vi "pulse_generator_multiheater_refnum.vi"(1 "125W Fixed/Variable":refnum<vi>, 2 "Stop! Refnum":refnum<vi>, 3 "Pulse Generator Control Multiheater Refnums":T1) -> ()   [LabVIEW 2015]
uses:
  <vilib>/Utility/error.llb/DialogType.ctl
  <vilib>/DAQmx/create/channels.llb/DAQmx Create Channel (DO-Digital Output).vi
  <vilib>/DAQmx/configure/timing.llb/DAQmx Timing (Implicit).vi
  <vilib>/DAQmx/create/channels.llb/DAQmx Create Channel (CO-Pulse Generation-Frequency).vi
  <resource>/objmgr/daqmx.rc
  <vilib>/DAQmx/write.llb/DAQmx Write (Digital 1D Bool NChan 1Samp 1Line).vi
  <vilib>/DAQmx/write.llb/DAQmx Write (Digital Bool 1Line 1Point).vi
  pulse_generator_controls_multiheater_refnums.ctl
panel:
  out "Stopped!":bool caption="OK"
  in  "Stop! Local":bool
  out "message":string=" INSTRUCTIONS:\r\rNormal Use:  When using subVIs that incorporate the error in/error out (or error I/O) structure, place this handler where you want to inform the user of an error, typically at the end of the I/O data path, as the last action of the program.  If the error in error? is ERROR, the handler creates a message describing the error and its source.  If the type of dialog = 1 (default), the message is displayed to the user, who can only acknowedge it.  If the type = 2, the user can acknowledge the message or abort execution; aborting a program with active I/O is not recommended.  If the type = 0, no message is displayed; this is used to process the error programmatically, and the error out cluster elements are wired to individual terminals for that reason.  \r\rOther Use:\n\r\nlocal testing.  To test the error code of a subVI or function that does not have the error I/O structure, you can wire its error code and a source string to the local error code and error source inputs.  If error in error? indicates no error and error code is not equal to 0, the local code and source are substituted for the error in values, and error? is set TRUE (ERROR)."
  in  "SwitchHelper":bool
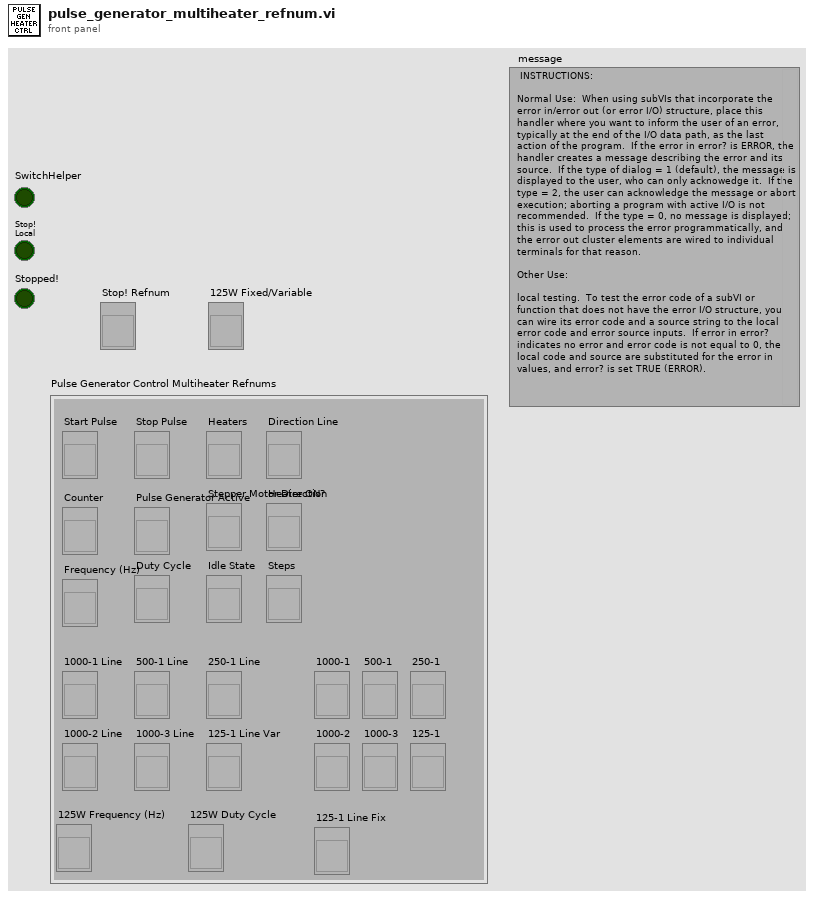
[diagram p1: front panel]
types:
  T1 = typedef "pulse_generator_controls_multiheater_refnums.ctl" = cluster{"Start Pulse":refnum<vi>, "Stop Pulse":refnum<vi>, "Heaters":refnum<vi>, "Counter":refnum<vi>, "Frequency (Hz)":refnum<vi>, "Duty Cycle":refnum<vi>, "Idle State":refnum<vi>, "Pulse Generator Active":refnum<vi>, "Stepper Motor Direction":refnum<vi>, "Steps":refnum<vi>, "Direction Line":refnum<vi>, "1000-1 Line":refnum<vi>, "1000-2 Line":refnum<vi>, "1000-3 Line":refnum<vi>, "500-1 Line":refnum<vi>, "250-1 Line":refnum<vi>, "125-1 Line Var":refnum<vi>, "1000-1":refnum<vi>, "1000-2":refnum<vi>, "1000-3":refnum<vi>, "500-1":refnum<vi>, "250-1":refnum<vi>, "125-1":refnum<vi>, "125W Frequency (Hz)":refnum<vi>, "125W Duty Cycle":refnum<vi>, "Heater ON?":refnum<vi>, "125-1 Line Fix":refnum<vi>}
  T2 = enum8{"Enabled", "Disabled", "Disabled and Grayed Out"}
  T3 = typedef "DialogType.ctl" = u16
  T4 = cluster{"1000-1":refnum<vi>, "1000-2":refnum<vi>, "1000-3":refnum<vi>, "500-1":refnum<vi>}
  T5 = cluster{"1000-1 Line":refnum<vi>, "1000-2 Line":refnum<vi>, "1000-3 Line":refnum<vi>, "500-1 Line":refnum<vi>, "250-1 Line":refnum<vi>}
  T6 = cluster{"1000-1 Line":refnum<vi>, "1000-2 Line":refnum<vi>, "1000-3 Line":refnum<vi>, "500-1 Line":refnum<vi>}
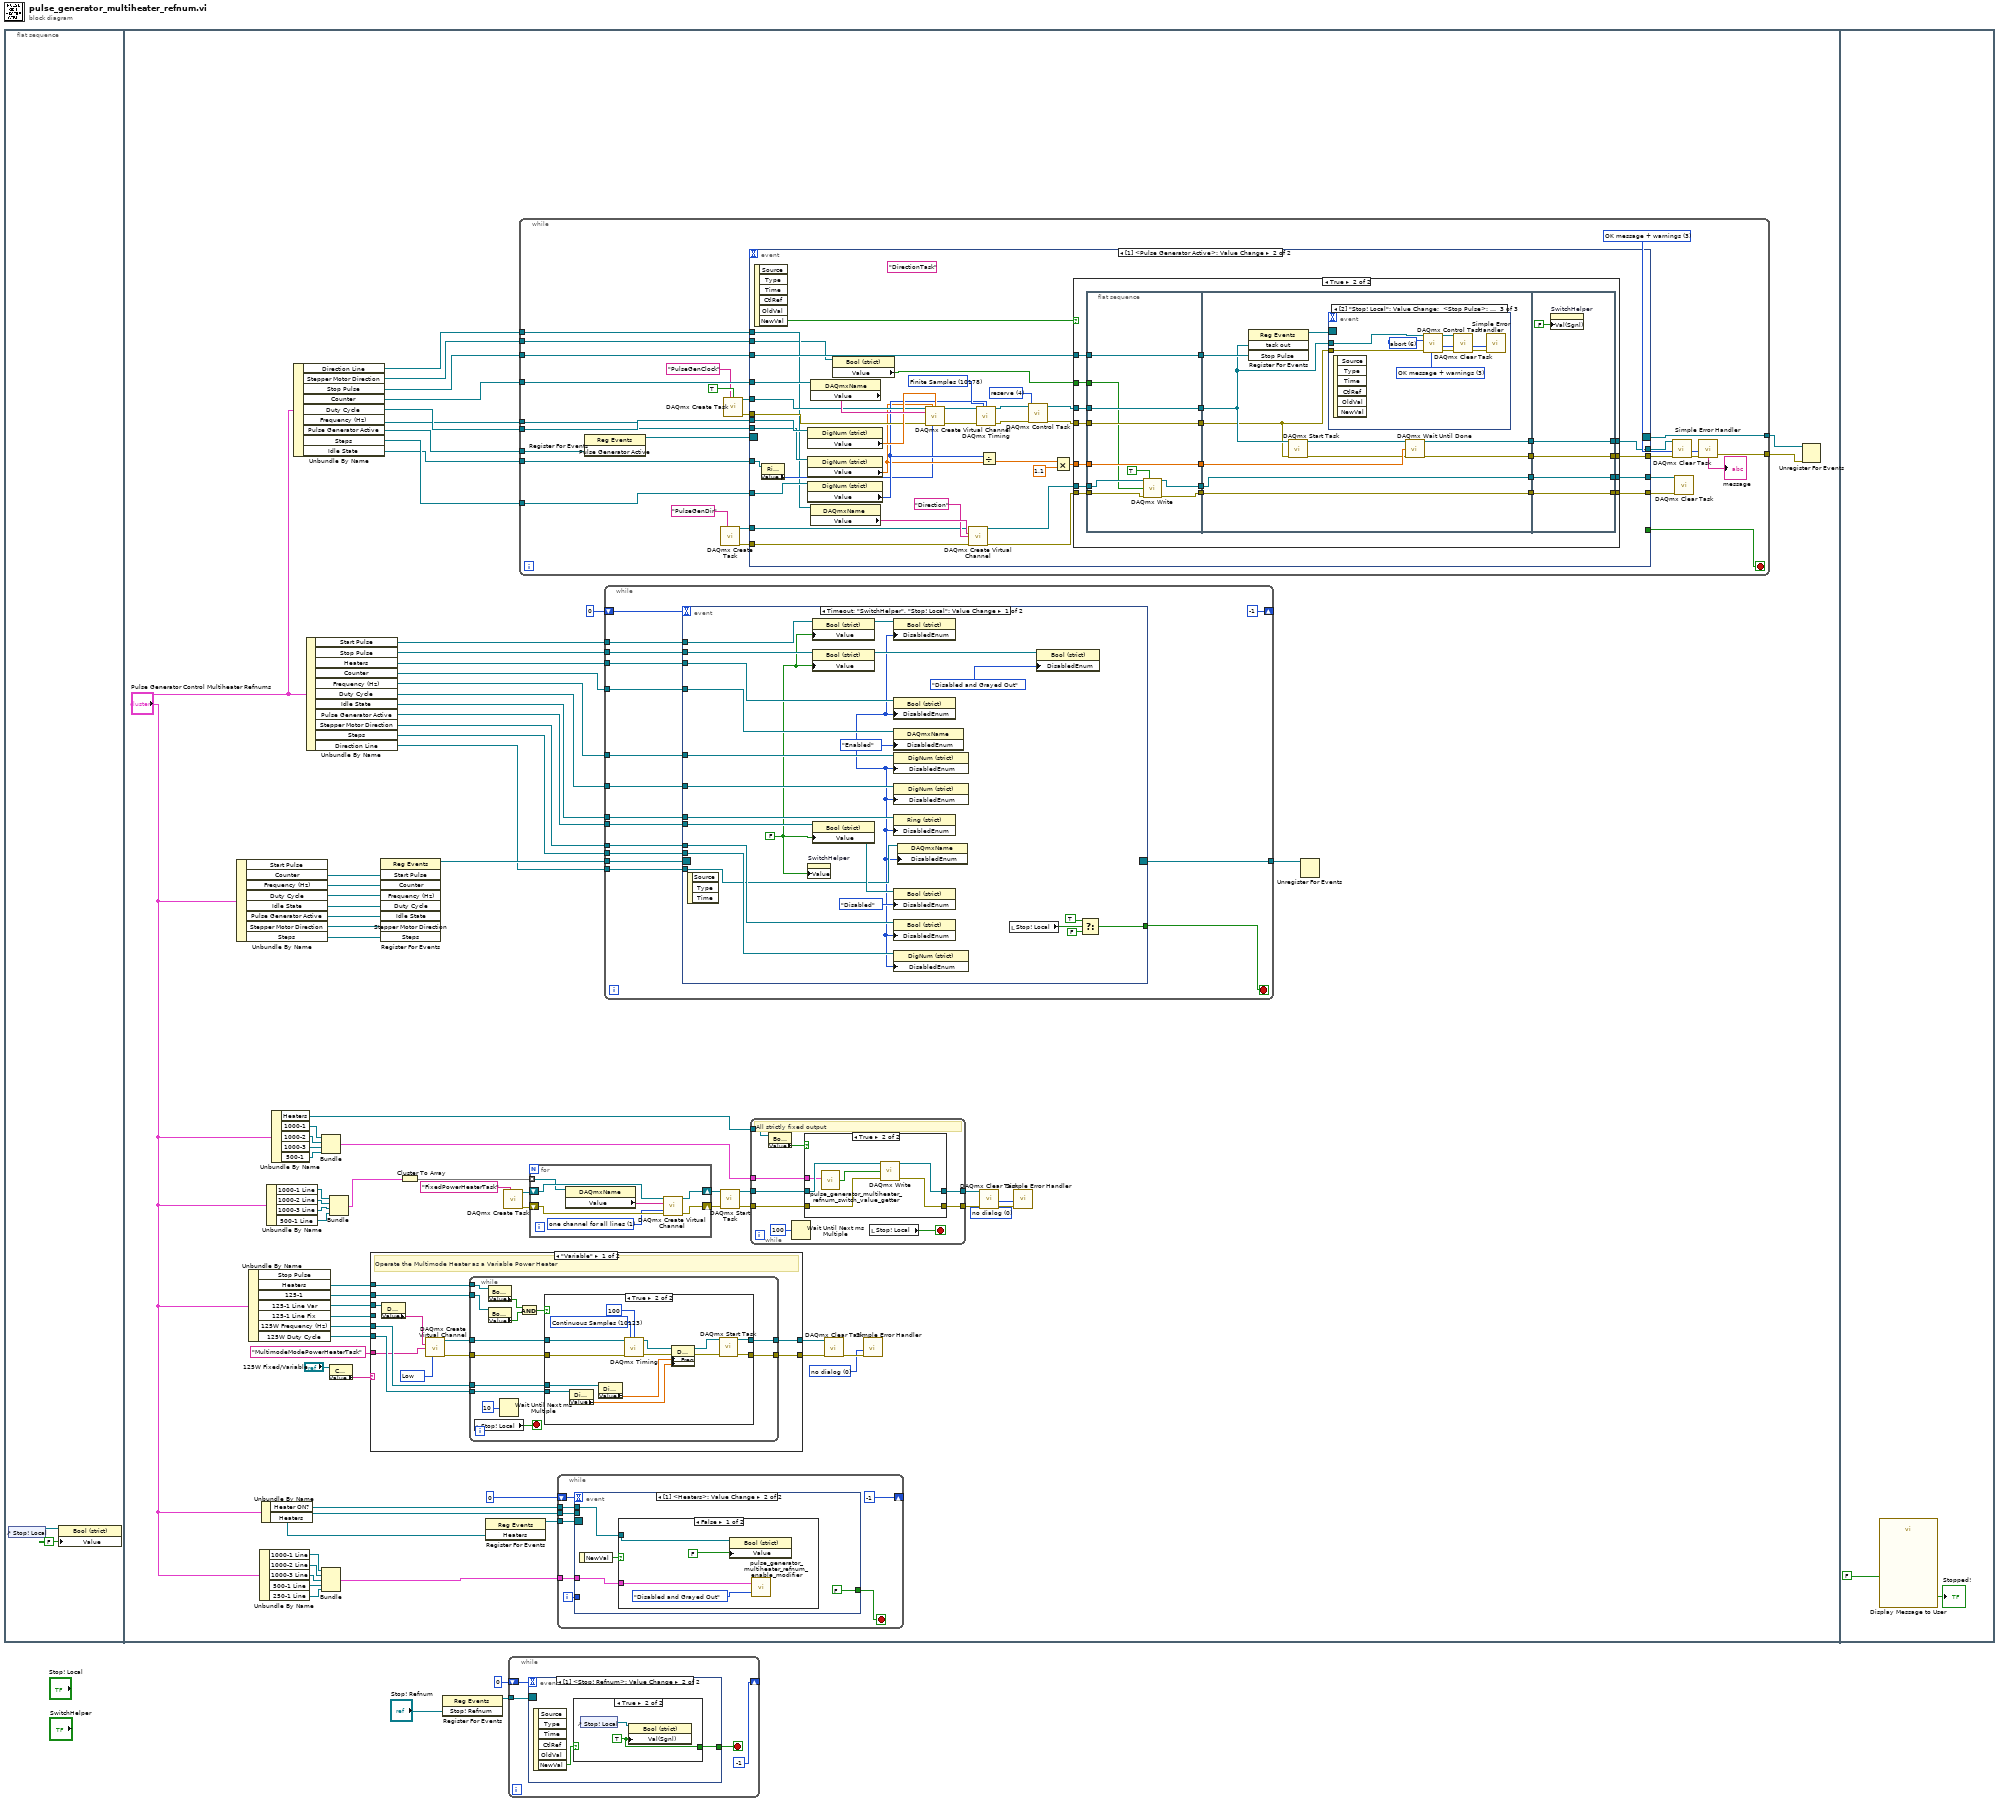
[diagram p0: block diagram]
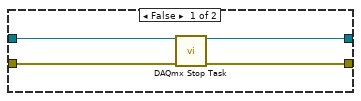
[diagram p2: hidden frame]
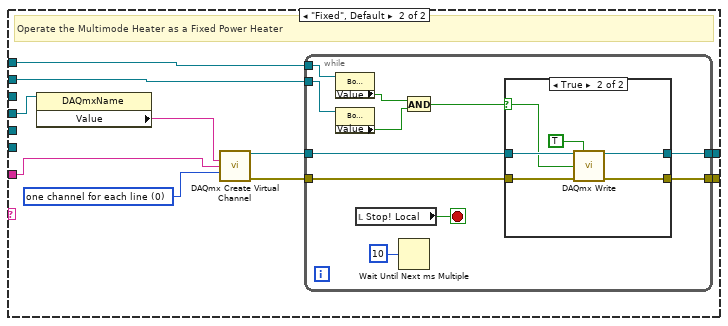
[diagram p3: hidden frame]
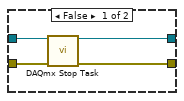
[diagram p4: hidden frame]
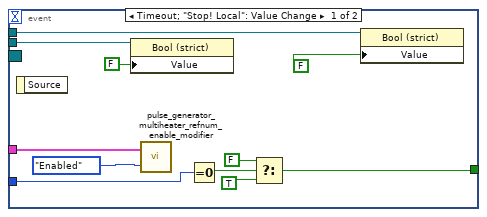
[diagram p5: hidden frame]
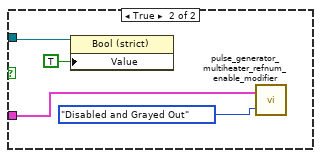
[diagram p6: hidden frame]
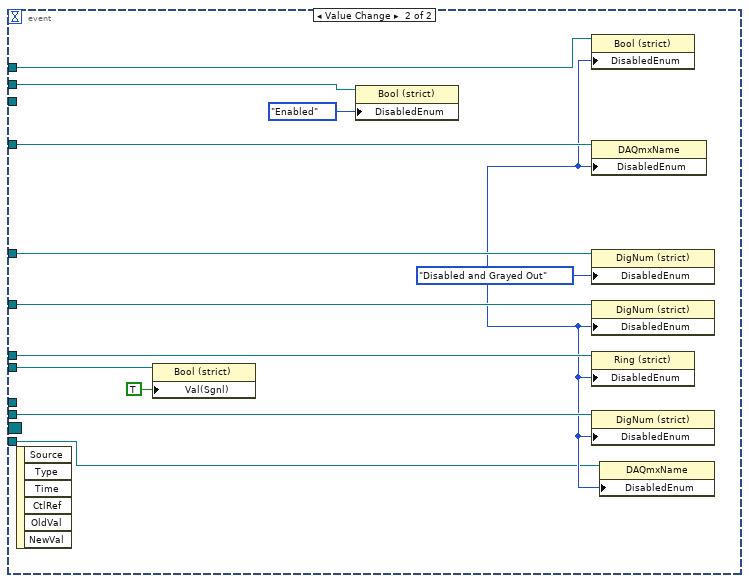
[diagram p8: hidden frame]
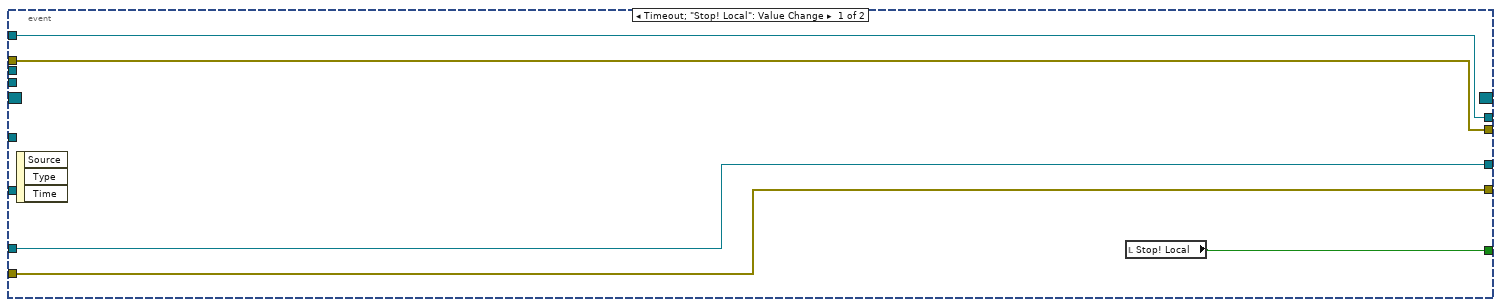
[diagram p9: hidden frame]
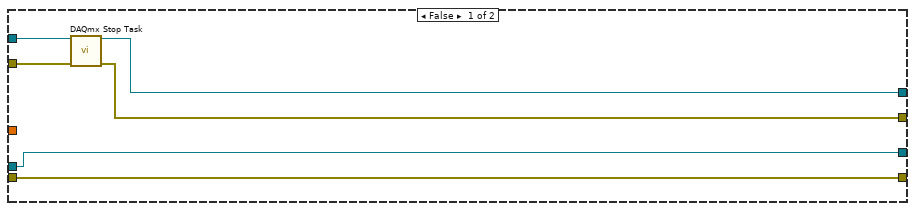
[diagram p10: hidden frame]
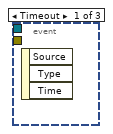
[diagram p11: hidden frame]
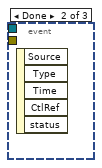
[diagram p12: hidden frame]
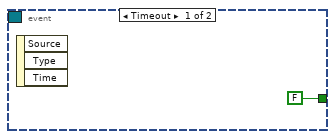
[diagram p13: hidden frame]
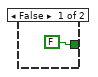
[diagram p14: hidden frame]
diagram:
  n1 = flat-sequence {
    frame #0 {
      n2 = control-ref of="Stop! Local"() -> (w4:refnum<vi>)
      n3 = property class="Bool (strict)"(reference=w4, "Value"=FALSE) -> ()  [unwired: 1 in, 2 out]
    }
    frame #1 {
      w7 = T3 0 items=["no dialog", "OK message", "continue or stop message", "OK message + warnings", "continue/stop + warnings"] ("type of dialog (OK msg:1)")
      w64 = T3 0 items=["no dialog", "OK message", "continue or stop message", "OK message + warnings", "continue/stop + warnings"] ("type of dialog (OK msg:1)")
      n4 = Unbundle By Name("Pulse Generator Control Multiheater Refnums") -> ("Start Pulse"=w73:refnum<vi>, "Counter"=w82:refnum<vi>, "Frequency (Hz)"=w81:refnum<vi>, "Duty Cycle"=w80:refnum<vi>, "Idle State"=w79:refnum<vi>, "Stepper Motor Direction"=w76:refnum<vi>, "Steps"=w75:refnum<vi>)  [unwired: 1 out]
      n5 = Unbundle By Name("Pulse Generator Control Multiheater Refnums") -> ("Heaters"=w14:refnum<vi>, "125-1"=w26:refnum<vi>, "125-1 Line Var"=w30:refnum<vi>, "125-1 Line Fix"=w8:refnum<vi>, "125W Frequency (Hz)"=w28:refnum<vi>, "125W Duty Cycle"=w27:refnum<vi>)  [unwired: 1 out]
      n6 = Unbundle By Name("Pulse Generator Control Multiheater Refnums") -> ("1000-1 Line"=w59:refnum<vi>, "1000-2 Line"=w58:refnum<vi>, "1000-3 Line"=w57:refnum<vi>, "500-1 Line"=w56:refnum<vi>, "250-1 Line"=w22:refnum<vi>)
      n7 = Unbundle By Name("Pulse Generator Control Multiheater Refnums") -> ("Heater ON?"=w62:refnum<vi>, "Heaters"=w50:refnum<vi>)
      n8 = Unbundle By Name("Pulse Generator Control Multiheater Refnums") -> ("1000-1 Line"=w20:refnum<vi>, "1000-2 Line"=w19:refnum<vi>, "1000-3 Line"=w18:refnum<vi>, "500-1 Line"=w17:refnum<vi>)
      n9 = Unbundle By Name("Pulse Generator Control Multiheater Refnums") -> ("Heaters"=w49:refnum<vi>, "1000-1"=w48:refnum<vi>, "1000-2"=w47:refnum<vi>, "1000-3"=w46:refnum<vi>, "500-1"=w45:refnum<vi>)
      n10 = Unbundle By Name("Pulse Generator Control Multiheater Refnums") -> ("Direction Line"=w12:refnum<vi>, "Stepper Motor Direction"=w11:refnum<vi>, "Stop Pulse"=w43:refnum<vi>, "Counter"=w39:refnum<vi>, "Duty Cycle"=w40:refnum<vi>, "Frequency (Hz)"=w37:refnum<vi>, "Pulse Generator Active"=w35:refnum<vi>, "Steps"=w33:refnum<vi>, "Idle State"=w29:refnum<vi>)
      n11 = Unbundle By Name("Pulse Generator Control Multiheater Refnums") -> ("Start Pulse"=w83:refnum<vi>, "Stop Pulse"=w42:refnum<vi>, "Heaters"=w60:refnum<vi>, "Counter"=w38:refnum<vi>, "Frequency (Hz)"=w36:refnum<vi>, "Duty Cycle"=w41:refnum<vi>, "Idle State"=w74:refnum<vi>, "Pulse Generator Active"=w34:refnum<vi>, "Stepper Motor Direction"=w66:refnum<vi>, "Steps"=w32:refnum<vi>, "Direction Line"=w13:refnum<vi>)
      n12 = Bundle("1000-1"=w48, "1000-2"=w47, "1000-3"=w46, "500-1"=w45) -> (w44:T4)  [unwired: 1 in]
      n13 = Bundle("1000-1 Line"=w59, "1000-2 Line"=w58, "1000-3 Line"=w57, "500-1 Line"=w56, "250-1 Line"=w22) -> (w16:T5)  [unwired: 1 in]
      n14 = Bundle("1000-1 Line"=w20, "1000-2 Line"=w19, "1000-3 Line"=w18, "500-1 Line"=w17) -> (w15:T6)  [unwired: 1 in]
      n15 = property class="CmbBox"(reference="125W Fixed/Variable") -> ("Value"=w9:string)  [unwired: 1 in, 2 out]
      n16 = case shown="\"Variable\"" w9 {
        tunnel: w30 -> [w96 _]
        tunnel: w28 -> [w91 _]
        tunnel: w27 -> [w90 _]
        tunnel: w26 -> [w89 w134]
        tunnel: [w88 w133] -> w24
        tunnel: [w87 w132] -> w23
        tunnel: w14 -> [w86 w131]
        tunnel: w8 -> [_ w130]
        tunnel: "MultimodeModePowerHeaterTask" ("new task name") -> [w85 w128]
        frame "Variable" {
          w94 = 10214 items=["High"=10192, "Low"=10214] ("idle state")
          # "Operate the Multimode Heater as a Variable Power Heater"
          n17 = property class="DAQmxName"(reference=w96) -> ("Value"=w95:string)  [unwired: 1 in, 2 out]
          n18 = call-poly <vilib>:"DAQmx Create Virtual Channel.vi"("counter"=w95, "name to assign"=w85, "idle state"=w94) -> ("task out"=w93:refnum<k21>, "error out"=w92:errorcluster)  [unwired: 11 in]
          n19 = while {
            tunnel: w93 -> [w107]
            tunnel: w92 -> [w106]
            tunnel: w89 -> [w101]
            tunnel: w91 -> [w105]
            tunnel: w90 -> [w104]
            tunnel: [w103] -> w88
            tunnel: [w102] -> w87
            tunnel: w86 -> [w100]
            stop <- w109 stop-if-true
            n20 = local read "Stop! Local"() -> (w109:bool)
            n21 = property class="Bool (strict)"(reference=w100) -> ("Value"=w98:bool)  [unwired: 1 in, 2 out]
            n22 = property class="Bool (strict)"(reference=w101) -> ("Value"=w97:bool)  [unwired: 1 in, 2 out]
            n23 = Wait Until Next ms Multiple(millisecond multiple=u32 10) -> ()  [unwired: 1 out]
            n24 = And(x=w98, y=w97) -> (x .and. y?=w99:bool)
            n25 = case shown="True" w99 {
              tunnel: w107 -> [w111 w127]
              tunnel: w106 -> [w110 w126]
              tunnel: w105 -> [_ w119]
              tunnel: w104 -> [_ w118]
              tunnel: [w113 w114] -> w103
              tunnel: [w112 w115] -> w102
              frame False {
                n26 = call <vilib>:"DAQmx Stop Task.vi"("task/channels in"=w111, "error in"=w110) -> ("task out"=w113:refnum<k21>, "error out"=w112:errorcluster)  [unwired: 12 in]
              }
              frame True {
                w125 = 10123 items=["Finite Samples"=10178, "Continuous Samples"=10123, "Hardware Timed Single Point"=12522] ("sample mode")
                n27 = property class="DigNum (strict)"(reference=w118) -> ("Value"=w120:dbl)  [unwired: 1 in, 2 out]
                n28 = property class="DigNum (strict)"(reference=w119) -> ("Value"=w121:dbl)  [unwired: 1 in, 2 out]
                n29 = call-poly <vilib>:"DAQmx Timing.vi"("task/channels in"=w127, "sample mode"=w125, "samples per channel"=100, "error in"=w126) -> ("task out"=w123:refnum<k21>, "error out"=w122:errorcluster)  [unwired: 10 in]
                n30 = property class="DAQmx Channel"(reference=w123, error in=w122, "CO.Pulse.Freq"=w121, "CO.Pulse.DutyCyc"=w120) -> (reference out=w117:refnum<k21>, error out=w116:errorcluster)
                n31 = call <vilib>:"DAQmx Start Task.vi"("task/channels in"=w117, "error in"=w116) -> ("task out"=w114:refnum<k21>, "error out"=w115:errorcluster)  [unwired: 12 in]
              }
            }
          }
        }
        frame "Fixed", Default {
          w129 = 0 items=["one channel for each line", "one channel for all lines"] ("line grouping")
          # "Operate the Multimode Heater as a Fixed Power Heater"
          n32 = property class="DAQmxName"(reference=w130) -> ("Value"=w137:string)  [unwired: 1 in, 2 out]
          n33 = call-poly <vilib>:"DAQmx Create Virtual Channel.vi"("lines"=w137, "name to assign"=w128, "line grouping"=w129) -> ("task out"=w136:refnum<k21>, "error out"=w135:errorcluster)  [unwired: 11 in]
          n34 = while {
            tunnel: w136 -> [w146]
            tunnel: w135 -> [w145]
            tunnel: w134 -> [w142]
            tunnel: [w144] -> w133
            tunnel: [w143] -> w132
            tunnel: w131 -> [w141]
            stop <- w148 stop-if-true
            n35 = property class="Bool (strict)"(reference=w141) -> ("Value"=w139:bool)  [unwired: 1 in, 2 out]
            n36 = property class="Bool (strict)"(reference=w142) -> ("Value"=w138:bool)  [unwired: 1 in, 2 out]
            n37 = local read "Stop! Local"() -> (w148:bool)
            n38 = Wait Until Next ms Multiple(millisecond multiple=u32 10) -> ()  [unwired: 1 out]
            n39 = And(x=w139, y=w138) -> (x .and. y?=w140:bool)
            n40 = case shown="True" w140 {
              selector: w140 -> [_ w153]
              tunnel: w146 -> [w150 w155]
              tunnel: w145 -> [w149 w154]
              tunnel: [w152 w158] -> w144
              tunnel: [w151 w157] -> w143
              frame False {
                n41 = call <vilib>:"DAQmx Stop Task.vi"("task/channels in"=w150, "error in"=w149) -> ("task out"=w152:refnum<k21>, "error out"=w151:errorcluster)  [unwired: 12 in]
              }
              frame True {
                n42 = call-poly <vilib>:"DAQmx Write.vi"("task/channels in"=w155, "auto start"=TRUE, "data"=w153, "error in"=w154) -> ("task out"=w158:refnum<k21>, "error out"=w157:errorcluster)  [unwired: 9 in, 1 out]
              }
            }
          }
        }
      }
      n43 = register-events(w73, w82, w81, w80, w79, w76, w75) -> (reference out=w78:refnum<event-registration>)  [unwired: 2 in, 1 out]
      n44 = Cluster To Array(cluster=w15) -> (array=w31:refnum<vi>[])
      n45 = register-events(w50) -> (reference out=w61:refnum<event-registration>)  [unwired: 2 in, 1 out]
      n46 = call <vilib>:"DAQmx Create Task.vi"("new task name"="FixedPowerHeaterTask") -> ("task out"=w53:refnum<k21>, "error out"=w52:errorcluster)  [unwired: 13 in]
      n47 = while {
        tunnel: w35 -> [w285]
        tunnel: [w287] -> w65
        tunnel: w33 -> [w280]
        tunnel: w40 -> [w278]
        tunnel: w37 -> [w275]
        tunnel: w39 -> [w279]
        tunnel: w43 -> [w286]
        tunnel: [w273] -> w63
        tunnel: w29 -> [w271]
        tunnel: w12 -> [w270]
        tunnel: w11 -> [w269]
        stop <- w274 stop-if-true
        w282 = T3 3 items=["no dialog", "OK message", "continue or stop message", "OK message + warnings", "continue/stop + warnings"] ("type of dialog (OK msg:1)")
        n48 = register-events(w285) -> (reference out=w284:refnum<event-registration>)  [unwired: 2 in, 1 out]
        n49 = call <vilib>:"DAQmx Create Task.vi"("new task name"="PulseGenDir") -> ("task out"=w268:refnum<k21>, "error out"=w267:errorcluster)  [unwired: 13 in]
        n50 = call <vilib>:"DAQmx Create Task.vi"("new task name"="PulseGenClock", "auto cleanup"=TRUE) -> ("task out"=w277:refnum<k21>, "error out"=w276:errorcluster)  [unwired: 12 in]
        n51 = event shown="[1] <Pulse Generator Active>: Value Change" {
          selector: w284 -> [_ _]
          dyn-events: [_ _] -> w287
          timeout: _ -> [_ _]
          tunnel: [w294 w331] -> w289
          tunnel: [w295 w332] -> w288
          tunnel: w277 -> [w295 w320]
          tunnel: w276 -> [w294 w319]
          tunnel: w286 -> [_ w330]
          tunnel: w280 -> [_ w325]
          tunnel: w279 -> [_ w323]
          tunnel: w278 -> [_ w321]
          tunnel: w275 -> [_ w316]
          tunnel: [w293 _] -> w274
          tunnel: w271 -> [_ w315]
          tunnel: w270 -> [_ w313]
          tunnel: w269 -> [_ w310]
          tunnel: w268 -> [w292 w308]
          tunnel: w267 -> [w291 w307]
          tunnel: [w292 w306] -> w266
          tunnel: [w291 w305] -> w265
          event Timeout; "Stop! Local": Value Change {
            n52 = event-data() -> ()  [unwired: 1 in, 3 out]
            n53 = local read "Stop! Local"() -> (w293:bool)
          }
          event Value Change {
            w302 = 4 items=["verify"=2, "reserve"=4, "commit"=3, "unreserve"=5, "abort"=6] ("action")
            (unwired) "DirectionTask" ("name to assign")
            w329 = 10178 items=["Finite Samples"=10178, "Continuous Samples"=10123, "Hardware Timed Single Point"=12522] ("sample mode")
            n54 = event-data() -> ("NewVal"=w333:bool)  [unwired: 1 in, 5 out]
            n55 = property class="Ring (strict)"(reference=w315) -> ("Value"=w314:i32)  [unwired: 1 in, 2 out]
            n56 = property class="DigNum (strict)"(reference=w321) -> ("Value"=w322:dbl)  [unwired: 1 in, 2 out]
            n57 = property class="DigNum (strict)"(reference=w316) -> ("Value"=w317:dbl)  [unwired: 1 in, 2 out]
            n58 = property class="DigNum (strict)"(reference=w325) -> ("Value"=w318:i32)  [unwired: 1 in, 2 out]
            n59 = property class="DAQmxName"(reference=w313) -> ("Value"=w312:string)  [unwired: 1 in, 2 out]
            n60 = property class="DAQmxName"(reference=w323) -> ("Value"=w324:string)  [unwired: 1 in, 2 out]
            n61 = property class="Bool (strict)"(reference=w310) -> ("Value"=w309:bool)  [unwired: 1 in, 2 out]
            n62 = call-poly <vilib>:"DAQmx Create Virtual Channel.vi"("task in"=w320, "frequency"=w317, "duty cycle"=w322, "counter"=w324, "error in"=w319, "idle state"=w314) -> ("task out"=w304:refnum<k21>, "error out"=w303:errorcluster)  [unwired: 8 in]
            n63 = call-poly <vilib>:"DAQmx Create Virtual Channel.vi"("task in"=w308, "lines"=w312, "name to assign"="Direction", "error in"=w307) -> ("task out"=w297:refnum<k21>, "error out"=w296:errorcluster)  [unwired: 10 in]
            n64 = call-poly <vilib>:"DAQmx Timing.vi"("task/channels in"=w304, "sample mode"=w329, "samples per channel"=w318, "error in"=w303) -> ("task out"=w301:refnum<k21>, "error out"=w300:errorcluster)  [unwired: 10 in]
            n65 = Divide(x=w318, y=w317) -> (x/y=w327:dbl)
            n66 = call <vilib>:"DAQmx Control Task.vi"("task/channels in"=w301, "action"=w302, "error in"=w300) -> ("task out"=w298:refnum<k21>, "error out"=w299:errorcluster)  [unwired: 11 in]
            n67 = Multiply(x=w327, y=1.1) -> (x*y=w326:dbl)
            n68 = case shown="True" w333 {
              tunnel: w298 -> [w339 w357]
              tunnel: w299 -> [w338 w360]
              tunnel: [w336 w359] -> w332
              tunnel: [w337 w358] -> w331
              tunnel: w330 -> [_ w354]
              tunnel: w326 -> [_ w353]
              tunnel: w309 -> [_ w352]
              tunnel: w297 -> [w335 w351]
              tunnel: w296 -> [w334 w350]
              tunnel: [w335 w348] -> w306
              tunnel: [w334 w346] -> w305
              frame False {
                n69 = call <vilib>:"DAQmx Stop Task.vi"("task/channels in"=w339, "error in"=w338) -> ("task out"=w336:refnum<k21>, "error out"=w337:errorcluster)  [unwired: 12 in]
              }
              frame True {
                n70 = flat-sequence {
                  tunnel: w350 -> [w365]
                  tunnel: w351 -> [w366]
                  tunnel: w352 -> [w361]
                  tunnel: w353 -> [w367]
                  tunnel: w354 -> [w368]
                  tunnel: w357 -> [w369]
                  tunnel: w360 -> [w370]
                  tunnel: [w370] -> w345
                  tunnel: [w369] -> w344
                  tunnel: [w368] -> w343
                  tunnel: [w367] -> w342
                  tunnel: [w364] -> w341
                  tunnel: [w363] -> w340
                  tunnel: [w381] -> w356
                  tunnel: [w380] -> w355
                  tunnel: [w371] -> w349
                  tunnel: [w372] -> w347
                  tunnel: w345 -> [w375]
                  tunnel: w344 -> [w376]
                  tunnel: w343 -> [w378]
                  tunnel: w342 -> [w377]
                  tunnel: w341 -> [w372]
                  tunnel: w340 -> [w371]
                  tunnel: [w392] -> w358
                  tunnel: [w393] -> w359
                  tunnel: w356 -> [w393]
                  tunnel: w355 -> [w392]
                  tunnel: w349 -> [w390]
                  tunnel: [w390] -> w348
                  tunnel: w347 -> [w389]
                  tunnel: [w389] -> w346
                  frame #0 {
                    n71 = call-poly <vilib>:"DAQmx Write.vi"("task/channels in"=w366, "auto start"=TRUE, "data"=w361, "error in"=w365) -> ("task out"=w363:refnum<k21>, "error out"=w364:errorcluster)  [unwired: 9 in, 1 out]
                  }
                  frame #1 {
                    n72 = register-events(w376, w378) -> (reference out=w379:refnum<event-registration>)  [unwired: 2 in, 1 out]
                    n73 = call <vilib>:"DAQmx Start Task.vi"("task/channels in"=w376, "error in"=w375) -> ("task out"=w374:refnum<k21>, "error out"=w373:errorcluster)  [unwired: 12 in]
                    n74 = event shown="[2] \"Stop! Local\": Value Change;  <Stop Pulse>: Value Change" {
                      selector: w379 -> [_ _ _]
                      dyn-events: _ -> [_ _ _]
                      timeout: _ -> [_ _ _]
                      tunnel: w376 -> [_ _ w388]
                      tunnel: w375 -> [_ _ w387]
                      event Timeout {
                        n75 = event-data() -> ()  [unwired: 1 in, 3 out]
                      }
                      event Done {
                        n76 = event-data() -> ()  [unwired: 1 in, 5 out]
                      }
                      event "Stop! Local": Value Change {
                        w382 = T3 3 items=["no dialog", "OK message", "continue or stop message", "OK message + warnings", "continue/stop + warnings"] ("type of dialog (OK msg:1)")
                        w386 = 6 items=["verify"=2, "reserve"=4, "commit"=3, "unreserve"=5, "abort"=6] ("action")
                        n77 = event-data() -> ()  [unwired: 1 in, 6 out]
                        n78 = call <vilib>:"DAQmx Control Task.vi"("task/channels in"=w388, "action"=w386, "error in"=w387) -> ("task out"=w385:refnum<k21>, "error out"=w384:errorcluster)  [unwired: 11 in]
                        n79 = call <vilib>:"DAQmx Clear Task.vi"("task in"=w385, "error in"=w384) -> ("error out"=w383:errorcluster)  [unwired: 13 in]
                        n80 = call <vilib>:"Simple Error Handler.vi"("type of dialog (OK msg:1)"=w382, "error in (no error)"=w383) -> ()  [unwired: 3 in, 5 out]
                      }
                    }
                    n81 = call <vilib>:"DAQmx Wait Until Done.vi"("task/channels in"=w374, "timeout (sec)"=w377, "error in"=w373) -> ("task out"=w381:refnum<k21>, "error out"=w380:errorcluster)  [unwired: 11 in]
                  }
                  frame #2 {
                    n82 = property on="SwitchHelper" class="Bool (strict)"("Val(Sgnl)"=FALSE ("Value (Signaling)")) -> ()  [unwired: 2 in, 2 out]
                  }
                }
              }
            }
          }
        }
        n83 = call <vilib>:"DAQmx Clear Task.vi"("task in"=w288, "error in"=w289) -> ("error out"=w290:errorcluster)  [unwired: 13 in]
        n84 = call <vilib>:"DAQmx Clear Task.vi"("task in"=w266, "error in"=w265) -> ()  [unwired: 13 in, 1 out]
        n85 = call <vilib>:"Simple Error Handler.vi"("type of dialog (OK msg:1)"=w282, "error in (no error)"=w290) -> ("error out"=w273:errorcluster, "message"=→"message":string)  [unwired: 3 in, 3 out]
      }
      n86 = for {
        tunnel: w31 -> [w161] mode=indexing
        shift-right: [w165] -> w55
        shift-left: w53 -> [w163]
        shift-right: [w164] -> w54
        shift-left: w52 -> [w162]
        w159 = 1 items=["one channel for each line", "one channel for all lines"] ("line grouping")
        n87 = property class="DAQmxName"(reference=w161) -> ("Value"=w160:string)  [unwired: 1 in, 2 out]
        n88 = call-poly <vilib>:"DAQmx Create Virtual Channel.vi"("task in"=w163, "lines"=w160, "line grouping"=w159, "error in"=w162) -> ("task out"=w165:refnum<k21>, "error out"=w164:errorcluster)  [unwired: 10 in]
      }
      n89 = while {
        tunnel: w61 -> [w173]
        shift-right: [-1 ("millisecond multiple")] -> _
        shift-left: 0 ("millisecond multiple") -> [w172]
        tunnel: w50 -> [w170]
        tunnel: w62 -> [w167]
        tunnel: w16 -> [w166]
        i -> [w169]
        stop <- w168 stop-if-true
        n90 = event shown="[1] <Heaters>: Value Change" {
          selector: w173 -> [_ _]
          dyn-events: _ -> [_ _]
          timeout: w172 -> [_ _]
          tunnel: w170 -> [w184 _]
          tunnel: w169 -> [w181 _]
          tunnel: [w178 FALSE ("f")] -> w168
          tunnel: w167 -> [w176 w187]
          tunnel: w166 -> [w175 w185]
          event Timeout; "Stop! Local": Value Change {
            n91 = event-data() -> ()  [unwired: 1 in, 1 out]
            n92 = property class="Bool (strict)"(reference=w184, "Value"=FALSE) -> ()  [unwired: 1 in, 2 out]
            n93 = call "pulse_generator_multiheater_refnum_enable_modifier.vi"("Disabled"=T2."Enabled", "DAQmxName Refnums"=w175) -> ()  [unwired: 1 in]
            n94 = Equal To 0?(x=w181) -> (x = 0?=w182:bool)
            n95 = Select(t=FALSE, s=w182, f=TRUE) -> (s? t:f=w178:bool)
            n96 = property class="Bool (strict)"(reference=w176, "Value"=FALSE) -> ()  [unwired: 1 in, 2 out]
          }
          event Value Change {
            n97 = event-data() -> ("NewVal"=w188:bool)  [unwired: 1 in]
            n98 = case shown="False" w188 {
              tunnel: w187 -> [w192 w195]
              tunnel: w185 -> [w190 w194]
              frame False {
                n99 = property class="Bool (strict)"(reference=w192, "Value"=FALSE) -> ()  [unwired: 1 in, 2 out]
                n100 = call "pulse_generator_multiheater_refnum_enable_modifier.vi"("Disabled"=T2."Disabled and Grayed Out", "DAQmxName Refnums"=w190) -> ()  [unwired: 1 in]
              }
              frame True {
                n101 = property class="Bool (strict)"(reference=w195, "Value"=TRUE) -> ()  [unwired: 1 in, 2 out]
                n102 = call "pulse_generator_multiheater_refnum_enable_modifier.vi"("Disabled"=T2."Disabled and Grayed Out", "DAQmxName Refnums"=w194) -> ()  [unwired: 1 in]
              }
            }
          }
        }
      }
      n103 = while {
        shift-right: [-1] -> _
        shift-left: 0 -> [w229]
        tunnel: w83 -> [w227]
        tunnel: w42 -> [w226]
        tunnel: w60 -> [w216]
        tunnel: w38 -> [w222]
        tunnel: w36 -> [w221]
        tunnel: w41 -> [w220]
        tunnel: w74 -> [w219]
        tunnel: w34 -> [w225]
        tunnel: w66 -> [w218]
        tunnel: w78 -> [w224]
        tunnel: [w223] -> w77
        tunnel: w32 -> [w217]
        tunnel: w13 -> [w214]
        stop <- w215 stop-if-true
        n104 = event shown="[0] Timeout;  \"SwitchHelper\", \"Stop! Local\": Value Change" {
          selector: w224 -> [_ _]
          dyn-events: [_ _] -> w223
          timeout: w229 -> [_ _]
          tunnel: w227 -> [w251 w263]
          tunnel: w226 -> [w250 w257]
          tunnel: w225 -> [w249 w255]
          tunnel: w222 -> [w238 w262]
          tunnel: w221 -> [w240 w258]
          tunnel: w220 -> [w242 w261]
          tunnel: w219 -> [w243 w260]
          tunnel: w218 -> [w237 _]
          tunnel: w217 -> [w241 w259]
          tunnel: w216 -> [w239 _]
          tunnel: [w234 _] -> w215
          tunnel: w214 -> [w231 w252]
          event Timeout; "SwitchHelper", "Stop! Local": Value Change {
            w230 = T2."Enabled" ("Disabled")
            w236 = FALSE ("Value")
            n105 = event-data() -> ()  [unwired: 1 in, 3 out]
            n106 = property on="SwitchHelper" class="Bool (strict)"("Value"=w236) -> ()  [unwired: 2 in, 2 out]
            n107 = property class="Bool (strict)"(reference=w251, "Value"=w236) -> (reference out=w248:refnum<vi>)  [unwired: 1 in, 1 out]
            n108 = property class="Bool (strict)"(reference=w250, "Value"=w236) -> (reference out=w247:refnum<vi>)  [unwired: 1 in, 1 out]
            n109 = property class="Bool (strict)"(reference=w249, "Value"=w236) -> (reference out=w246:refnum<vi>)  [unwired: 1 in, 1 out]
            n110 = property class="Bool (strict)"(reference=w248, "DisabledEnum"=w230) -> ()  [unwired: 1 in, 2 out]
            n111 = property class="Bool (strict)"(reference=w239, "DisabledEnum"=w230) -> ()  [unwired: 1 in, 2 out]
            n112 = property class="DAQmxName"(reference=w238, "DisabledEnum"=w230) -> ()  [unwired: 1 in, 2 out]
            n113 = property class="DigNum (strict)"(reference=w240, "DisabledEnum"=w230) -> ()  [unwired: 1 in, 2 out]
            n114 = property class="DigNum (strict)"(reference=w242, "DisabledEnum"=w230) -> ()  [unwired: 1 in, 2 out]
            n115 = property class="Ring (strict)"(reference=w243, "DisabledEnum"=w230) -> ()  [unwired: 1 in, 2 out]
            n116 = property class="Bool (strict)"(reference=w246, "DisabledEnum"=T2."Disabled" ("Disabled")) -> ()  [unwired: 1 in, 2 out]
            n117 = property class="Bool (strict)"(reference=w237, "DisabledEnum"=w230) -> ()  [unwired: 1 in, 2 out]
            n118 = property class="DigNum (strict)"(reference=w241, "DisabledEnum"=w230) -> ()  [unwired: 1 in, 2 out]
            n119 = property class="DAQmxName"(reference=w231, "DisabledEnum"=w230) -> ()  [unwired: 1 in, 2 out]
            n120 = local read "Stop! Local"() -> (w235:bool)
            n121 = property class="Bool (strict)"(reference=w247, "DisabledEnum"=T2."Disabled and Grayed Out" ("Disabled")) -> ()  [unwired: 1 in, 2 out]
            n122 = Select(t=TRUE ("Value"), s=w235, f=FALSE ("Value")) -> (s? t:f=w234:bool)
          }
          event Value Change {
            w253 = T2."Disabled and Grayed Out" ("Disabled")
            n123 = event-data() -> ()  [unwired: 1 in, 6 out]
            n124 = property class="Bool (strict)"(reference=w255, "Val(Sgnl)"=TRUE ("Value")) -> ()  [unwired: 1 in, 2 out]
            n125 = property class="Bool (strict)"(reference=w257, "DisabledEnum"=T2."Enabled" ("Disabled")) -> ()  [unwired: 1 in, 2 out]
            n126 = property class="Bool (strict)"(reference=w263, "DisabledEnum"=w253) -> ()  [unwired: 1 in, 2 out]
            n127 = property class="DAQmxName"(reference=w262, "DisabledEnum"=w253) -> ()  [unwired: 1 in, 2 out]
            n128 = property class="DigNum (strict)"(reference=w258, "DisabledEnum"=w253) -> ()  [unwired: 1 in, 2 out]
            n129 = property class="DigNum (strict)"(reference=w261, "DisabledEnum"=w253) -> ()  [unwired: 1 in, 2 out]
            n130 = property class="Ring (strict)"(reference=w260, "DisabledEnum"=w253) -> ()  [unwired: 1 in, 2 out]
            n131 = property class="DigNum (strict)"(reference=w259, "DisabledEnum"=w253) -> ()  [unwired: 1 in, 2 out]
            n132 = property class="DAQmxName"(reference=w252, "DisabledEnum"=w253) -> ()  [unwired: 1 in, 2 out]
          }
        }
      }
      n133 = call <vilib>:"DAQmx Start Task.vi"("task/channels in"=w55, "error in"=w54) -> ("task out"=w71:refnum<k21>, "error out"=w72:errorcluster)  [unwired: 12 in]
      n134 = while {
        tunnel: w71 -> [w203]
        tunnel: w72 -> [w202]
        tunnel: w49 -> [w198]
        tunnel: [w201] -> w70
        tunnel: [w200] -> w69
        tunnel: w44 -> [w199]
        stop <- w204 stop-if-true
        # "All strictly fixed output"
        n135 = property class="Bool (strict)"(reference=w198) -> ("Value"=w197:bool)  [unwired: 1 in, 2 out]
        n136 = Wait Until Next ms Multiple(millisecond multiple=u32 100) -> ()  [unwired: 1 out]
        n137 = case shown="True" w197 {
          tunnel: w203 -> [w207 w212]
          tunnel: w202 -> [w206 w209]
          tunnel: [w207 w213] -> w201
          tunnel: [w206 w208] -> w200
          tunnel: w199 -> [_ w211]
          frame False {
          }
          frame True {
            n138 = call "pulse_generator_multiheater_refnum_switch_value_getter.vi"("output cluster"=w211) -> ("Array"=w210:bool[])
            n139 = call-poly <vilib>:"DAQmx Write.vi"("task/channels in"=w212, "data"=w210, "error in"=w209) -> ("task out"=w213:refnum<k21>, "error out"=w208:errorcluster)  [unwired: 10 in, 1 out]
          }
        }
        n140 = local read "Stop! Local"() -> (w204:bool)
      }
      n141 = call <vilib>:"DAQmx Clear Task.vi"("task in"=w24, "error in"=w23) -> ("error out"=w25:errorcluster)  [unwired: 13 in]
      n142 = call <vilib>:"Simple Error Handler.vi"("type of dialog (OK msg:1)"=w7, "error in (no error)"=w25) -> ()  [unwired: 3 in, 5 out]
      n143 = call <vilib>:"DAQmx Clear Task.vi"("task in"=w70, "error in"=w69) -> ("error out"=w68:errorcluster)  [unwired: 13 in]
      n144 = call <vilib>:"Simple Error Handler.vi"("type of dialog (OK msg:1)"=w64, "error in (no error)"=w68) -> ()  [unwired: 3 in, 5 out]
      n145 = Unregister For Events(event registration refnum=w77) -> ()  [unwired: 1 in, 1 out]
      n146 = Unregister For Events(event registration refnum=w65, error in=w63) -> ()  [unwired: 1 out]
    }
    frame #2 {
      n147 = call "Display Message to User"("Enable"=FALSE) -> ("OK"=→"Stopped!":bool)  [unwired: 9 in, 1 out]
    }
  }
  n148 = register-events("Stop! Refnum") -> (reference out=w2:refnum<event-registration>)  [unwired: 2 in, 1 out]
  n149 = while {
    tunnel: w2 -> [w399]
    shift-right: [-1] -> _
    shift-left: 0 -> [w398]
    stop <- w396 stop-if-true
    n150 = event shown="[1] <Stop! Refnum>: Value Change" {
      selector: w399 -> [_ _]
      dyn-events: _ -> [_ _]
      timeout: w398 -> [_ _]
      tunnel: [FALSE ("Value (Signaling)") w401] -> w396
      event Timeout {
        n151 = event-data() -> ()  [unwired: 1 in, 3 out]
      }
      event Value Change {
        n152 = event-data() -> ("NewVal"=w402:bool)  [unwired: 1 in, 5 out]
        n153 = case shown="True" w402 {
          tunnel: [FALSE ("Value (Signaling)") w405] -> w401
          frame False {
          }
          frame True {
            w405 = TRUE ("Value (Signaling)")
            n154 = control-ref of="Stop! Local"() -> (w404:refnum<vi>)
            n155 = property class="Bool (strict)"(reference=w404, "Val(Sgnl)"=w405) -> ()  [unwired: 1 in, 2 out]
          }
        }
      }
    }
  }
